vi "XML - Remove Old Tx Channels.vi"(8 "error in (no error)":errorcluster, 11 "Device Item Ref in":T1 format="%.0x") -> (0 "error out":errorcluster, 2 "Tx Dependent Refs":T1[](array[typedef]) format="%.0x", 3 "Device Item Ref out":T1 format="%.0x")   [LabVIEW 2019]
uses:
  <vilib>/NI VeriStand/Custom Device API/Custom Device Item Ref.ctl
  Shared/Constants.vi
  <vilib>/NI VeriStand/Custom Device Tools/Custom Device Utility Library/NI VeriStand - Search for Item by GUID.vi
  <vilib>/NI VeriStand/Custom Device Tools/Custom Device Utility Library/Custom Device Utility Library.lvlib
  <vilib>/NI VeriStand/Custom Device API/Custom Device API.lvlib
  Shared/UDP-Custom-Device Shared.lvlib
  Property Accessors/Shared Packet Accessors.lvlib
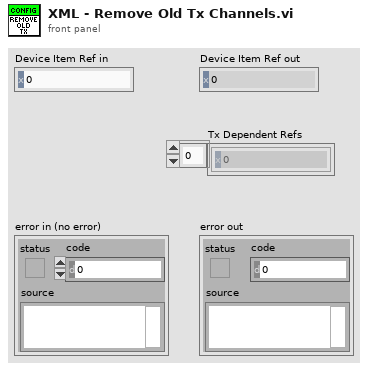
[diagram p1: front panel]
types:
  T1 = typedef "Custom Device API.lvlib/Custom Device Item Ref.ctl" = u64
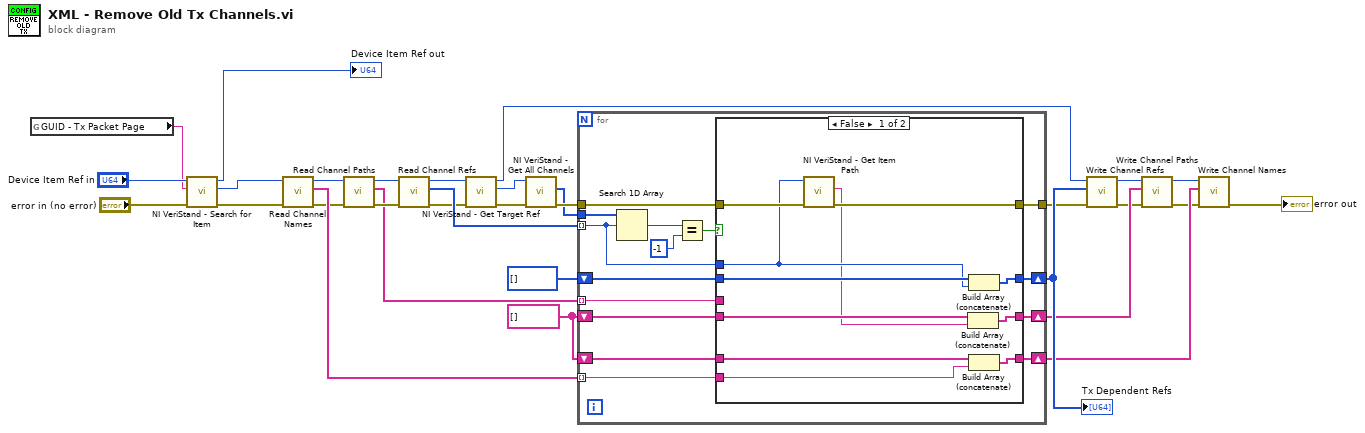
[diagram p0: block diagram]
diagram:
  w29 = string[] []
  n1 = global read "Constants.vi" "GUID - Tx Packet Page"() -> (w22:string)
  n2 = call-poly <vilib>:"NI VeriStand - Search for Item.vi"("error in"="error in (no error)", "Item GUID"=w22, "Section Ref in"="Device Item Ref in") -> ("error out"=w17:errorcluster, "Item Ref"=w18:T1, "Section Ref out"=→"Device Item Ref out":T1)  [unwired: 5 in, 1 out]
  n3 = call "Read Channel Names.vi"("error in (no error)"=w17, "Node Ptr"=w18) -> ("error out"=w14:errorcluster, "Channel Names"=w16:string[], "Node Ptr out"=w15:T1)  [unwired: 7 in]
  n4 = call "Read Channel Paths.vi"("error in (no error)"=w14, "Node Ptr"=w15) -> ("error out"=w12:errorcluster, "Channel Paths"=w11:string[], "Node Ptr out"=w13:T1)  [unwired: 7 in]
  n5 = call "Read Channel Refs.vi"("error in (no error)"=w12, "Node Ptr"=w13) -> ("error out"=w20:errorcluster, "Dependent Node Refs"=w21:T1[], "Node Ptr out"=w19:T1)  [unwired: 7 in]
  n6 = call <vilib>:"NI VeriStand - Get Target Ref.vi"("error in"=w20, "Item Ref in"=w19) -> ("error out"=w25:errorcluster, "Target Ref"=w26:T1, "Item Ref out"=w10:T1)  [unwired: 6 in, 1 out]
  n7 = call <vilib>:"NI VeriStand - Get All Channels.vi"("error in"=w25, "Section Ref in"=w26) -> ("error out"=w28:errorcluster, "Channel Refs"=w27:T1[])  [unwired: 6 in, 2 out]
  n8 = for {
    tunnel: w27 -> [w46]
    tunnel: w21 -> [w33] mode=indexing
    tunnel: w28 -> [w42]
    tunnel: w16 -> [w41] mode=indexing
    tunnel: w11 -> [w40] mode=indexing
    shift-right: [w35] -> w6
    shift-left: w29 -> [w38]
    shift-right: [w34] -> w4
    shift-left: w29 -> [w39]
    shift-right: [w36] -> w9
    shift-left: T1[] [] -> [w37]
    tunnel: [w32] -> w8
    n9 = Search 1D Array(1D array=w46, element=w33) -> (index of element=w45:i32)  [unwired: 1 in]
    n10 = Equal?(x=w45, y=-1) -> (x = y?=w43:bool)
    n11 = case shown="False" w43 {
      tunnel: w42 -> [w50 w58]
      tunnel: w41 -> [w52 _]
      tunnel: w40 -> [_ _]
      tunnel: w39 -> [w53 w59]
      tunnel: w38 -> [w55 w60]
      tunnel: w37 -> [w57 w61]
      tunnel: [w56 w61] -> w36
      tunnel: [w54 w60] -> w35
      tunnel: [w51 w59] -> w34
      tunnel: w33 -> [w48 _]
      tunnel: [w49 w58] -> w32
      frame False {
        n12 = call <vilib>:"NI VeriStand - Get Item Path.vi"("error in (no error)"=w50, "Item Ref in"=w48) -> ("error out"=w49:errorcluster, "Path"=w47:string)  [unwired: 6 in, 2 out]
        n13 = Build Array (concatenate)(w55, w47) -> (w54:string[])
        n14 = Build Array (concatenate)(w57, w48) -> (w56:T1[])
        n15 = Build Array (concatenate)(w53, w52) -> (w51:string[])
      }
      frame True {
      }
    }
  }
  "Tx Dependent Refs" <- w9
  n16 = call "Write Channel Refs.vi"("error in (no error)"=w8, "Dependent Node Refs"=w9, "Node Ptr"=w10) -> ("error out"=w3:errorcluster, "Node Ptr out"=w7:T1)  [unwired: 7 in]
  n17 = call "Write Channel Paths.vi"("error in (no error)"=w3, "Channel Paths"=w6, "Node Ptr"=w7) -> ("error out"=w2:errorcluster, "Node Ptr out"=w5:T1)  [unwired: 7 in]
  n18 = call "Write Channel Names.vi"("error in (no error)"=w2, "Channel Names"=w4, "Node Ptr"=w5) -> ("error out"=→"error out":errorcluster)  [unwired: 7 in, 1 out]
